vi "Configure External Logging.vi"(0 "VISA resource name":refnum<visa-resource-name>, 1 "Enable Voltage Measurements (False)":bool, 2 "Enable Current Measurements (False)":bool, 5 "Auto Range (True)":bool=TRUE, 7 "Manual Range (0)":dbl, 9 "Logging Period (60)":dbl=60.0, 11 "error in (no error)":errorcluster, 12 "Enable Voltage Extrema Measurement (False)":bool, 13 "Enable Current Extrema Measurement (False)":bool) -> (4 "VISA resource name out":refnum<visa-resource-name>, 15 "error out":errorcluster)   [LabVIEW 2021, in "Agilent N6900 N7900 Series.lvlib"]
doc: "Configures what settings are useful for configuring external logging.\n\nNote: Only valid in the N7900 series"
uses:
  <instrlib>/Agilent N6900 N7900 Series/Agilent N6900 N7900 Series.lvlib
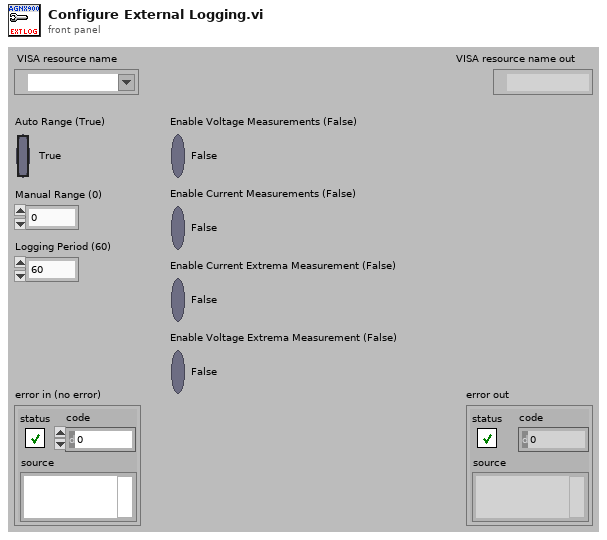
[diagram p1: front panel]
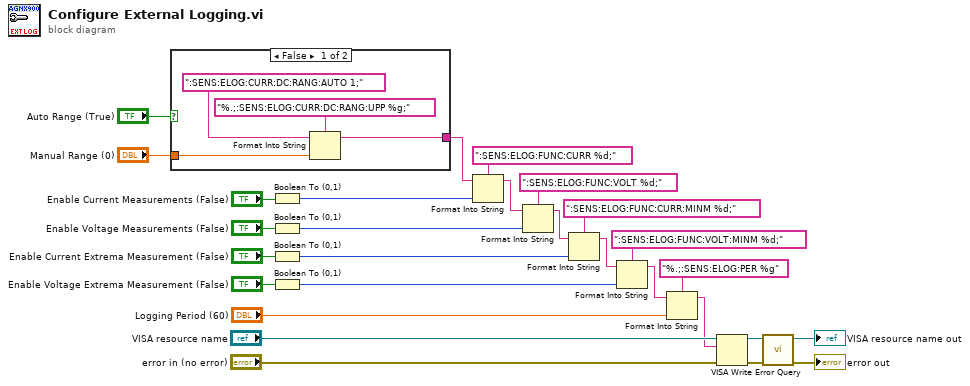
[diagram p0: block diagram]
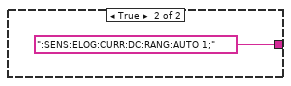
[diagram p2: hidden frame]
diagram:
  n1 = case shown="False" "Auto Range (True)" {
    tunnel: "Manual Range (0)" -> [w30 _]
    tunnel: [w32 ":SENS:ELOG:CURR:DC:RANG:AUTO 1;"] -> w2
    frame False {
      n2 = Format Into String(format string="%.;:SENS:ELOG:CURR:DC:RANG:UPP %g;", initial string=":SENS:ELOG:CURR:DC:RANG:AUTO 1;", w30) -> (resulting string=w32:string)  [unwired: 1 in, 1 out]
    }
    frame True {
    }
  }
  n3 = Boolean To (0,1)(Boolean="Enable Current Measurements (False)") -> (0, 1=w6:i16)
  n4 = Boolean To (0,1)(Boolean="Enable Voltage Measurements (False)") -> (0, 1=w9:i16)
  n5 = Boolean To (0,1)(Boolean="Enable Current Extrema Measurement (False)") -> (0, 1=w13:i16)
  n6 = Boolean To (0,1)(Boolean="Enable Voltage Extrema Measurement (False)") -> (0, 1=w17:i16)
  n7 = Format Into String(format string=":SENS:ELOG:FUNC:CURR %d;", initial string=w2, w6) -> (resulting string=w1:string)  [unwired: 1 in, 1 out]
  n8 = Format Into String(format string=":SENS:ELOG:FUNC:VOLT %d;", initial string=w1, w9) -> (resulting string=w8:string)  [unwired: 1 in, 1 out]
  n9 = Format Into String(format string=":SENS:ELOG:FUNC:CURR:MINM %d;", initial string=w8, w13) -> (resulting string=w14:string)  [unwired: 1 in, 1 out]
  n10 = Format Into String(format string=":SENS:ELOG:FUNC:VOLT:MINM %d;", initial string=w14, w17) -> (resulting string=w19:string)  [unwired: 1 in, 1 out]
  n11 = Format Into String(format string="%.;:SENS:ELOG:PER %g", initial string=w19, "Logging Period (60)") -> (resulting string=w22:string)  [unwired: 1 in, 1 out]
  n12 = VISA Write(VISA resource name="VISA resource name", write buffer=w22, error in (no error)="error in (no error)") -> (VISA resource name out=w25:refnum<visa-resource-name>, error out=w26:errorcluster)  [unwired: 1 out]
  n13 = call <instrlib>:"Error Query.vi"("error in (no error)"=w26, "VISA resource name"=w25) -> ("error out"=→"error out":errorcluster, "VISA resource name out"=→"VISA resource name out":refnum<visa-resource-name>)  [unwired: 6 in, 2 out]
